vi "Process.vi"(8 "error in":errorcluster, 11 "Instrument":refnum<class "Instrument.lvclass">) -> (0 "error out":errorcluster, 3 "Instrument out":refnum<class "Instrument.lvclass">)   [LabVIEW 2016, in "Instrument.lvclass"]
doc: "---------------------------------------------------------------\nJKI State Machine Objects™\nhttp://jki.net/state-machine-objects/\nCopyright (C) 2005-2015, JKI <info@jki.net>\nALL RIGHTS RESERVED"
uses:
  Instrument.lvclass
  C:/Program Files (x86)/National Instruments/LabVIEW 2016/vi.lib/JKI/JKI SMO/SMO/SMO.lvclass
  <vilib>/JKI/JKI SMO/SMO/Typedefs/Parent Call--Enum.ctl
  RemoteControl/Typedefs/Message--Cluster.ctl
  RemoteControl/Typedefs/PrivateEvents--RemoteControl.Configure.ctl
  Logger.PGSQL/Typedefs/PrivateEvents--Logger.PGSQL.Write Variable.ctl
  <vilib>/JKI/JKI SMO/SMO/Typedefs/Public Events.ctl
  <vilib>/JKI/JKI SMO/SMO/Typedefs/SMOState --Enum.ctl
  <vilib>/JKI/JKI SMO/SMO/Typedefs/Reserve State--Enum.ctl
  RemoteControl/Typedefs/PrivateEvents--RemoteControl.SendMessageToProcess.ctl
  RemoteControl/RemoteControl.lvclass
  Logger.Error/Logger.Error.lvclass
  Logger.PGSQL/Logger.PGSQL.lvclass
  <vilib>/JKI/JKI SMO/SMO/SMO.lvclass
panel:
  out "Local Command":string
  out "Name":string
  out "Remote Command":string
  # "1. Receives & processes commands from RemoteControl process\n2. Logs instrument settings to DSC using Logger process"
  # "INSTRUMENT"
  # "For instructions on how to use the JKI State Machine Objects, examples and video tutorials, visit:\nhttp://jki.net/state-machine-objects/\n\nJKI State Machine Objects™\nhttp://jki.net/state-machine-objects/\nCopyright (C) 2005-2015, JKI <info@jki.net>\nALL RIGHTS RESERVED"
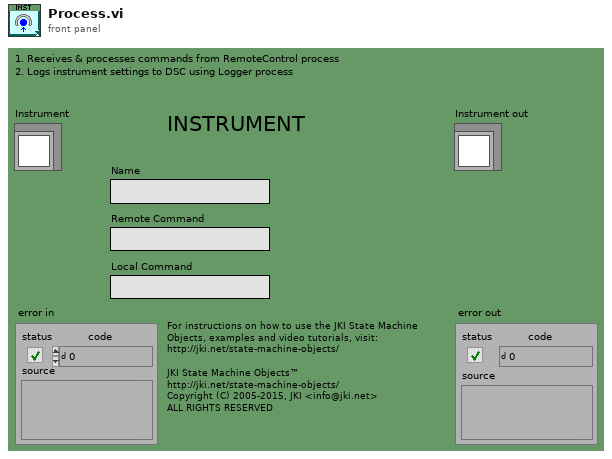
[diagram p1: front panel]
types:
  T1 = typedef "SMO.lvclass/Parent Call--Enum.ctl" = enum16{"Allows parent to run", "Does not request parent to run"}
  T2 = enum32{"invalid app kind", "Development System", "Run Time System", "Student Edition", "Embedded LabVIEW", "Evaluation", "Custom"}
  T3 = enum32{"Invalid", "Standard", "Closed", "Hidden", "Minimized", "Maximized"}
  T4 = enum32{"Bad", "Idle", "Run top level", "Running"}
  T5 = typedef "RemoteControl.lvclass/PrivateEvents--RemoteControl.SendMessageToProcess.ctl" = cluster{"Message":T6}
  T6 = typedef "RemoteControl.lvclass/Message--Cluster.ctl" = cluster{"Command":string, "Data":variant, "Message ID":i32}
  T7 = typedef "Instrument.lvclass/Dependencies--Cluster.ctl" = cluster{"RemoteControl":refnum<class "RemoteControl.lvclass">, "Logger.Error":refnum<class "Logger.Error.lvclass">, "Logger.PGSQL":refnum<class "Logger.PGSQL.lvclass">}
  T8 = typedef "RemoteControl.lvclass/PrivateEvents--RemoteControl.Configure.ctl" = cluster{"address":string, "Port":u16, "AllowedRemote":string, "Commands":string[]}
  T9 = typedef "Logger.PGSQL.lvclass/PrivateEvents--Logger.PGSQL.Write Variable.ctl" = cluster{"Address":string, "Data":variant}
  T10 = cluster{"Core":cluster{"Current VI Reference":refnum<vi>, "Close Panel on Exit?":bool, "error":errorcluster}, "Self Reference":refnum<class "Instrument.lvclass">, "Dependencies":T7, "RC Configuration":T8, "Message":T6, "getAll":variant, "Debug Mode?":bool, "PGSQL":T9}
  T11 = typedef "SMO.lvclass/SMOState --Enum.ctl" = enum16{"unknown", "Created", "Started", "Stopped"}
  T12 = cluster{"Current VI Reference":refnum<vi>, "Close Panel on Exit?":bool, "error":errorcluster}
  T13 = typedef "SMO.lvclass/Public Events.ctl" = cluster{"Error":refnum<user-event>, "State":refnum<user-event>, "Reserve State":refnum<user-event>}
  T14 = typedef "SMO.lvclass/Protected Events.ctl" = cluster{"StopProcesses":refnum<user-event>, "AbortProcesses":refnum<user-event>, "Config Changed":refnum<user-event>, "Dependency":refnum<user-event>}
  T15 = typedef "RemoteControl.lvclass/PublicEvents--Cluster.ctl" = cluster{"SendMessageFromProcess":refnum<user-event>}
  T16 = typedef "Instrument.lvclass/PrivateEvents--Cluster.ctl" = cluster{"MessageToProcess":refnum<user-event>, "Log PGSQL":refnum<user-event>}
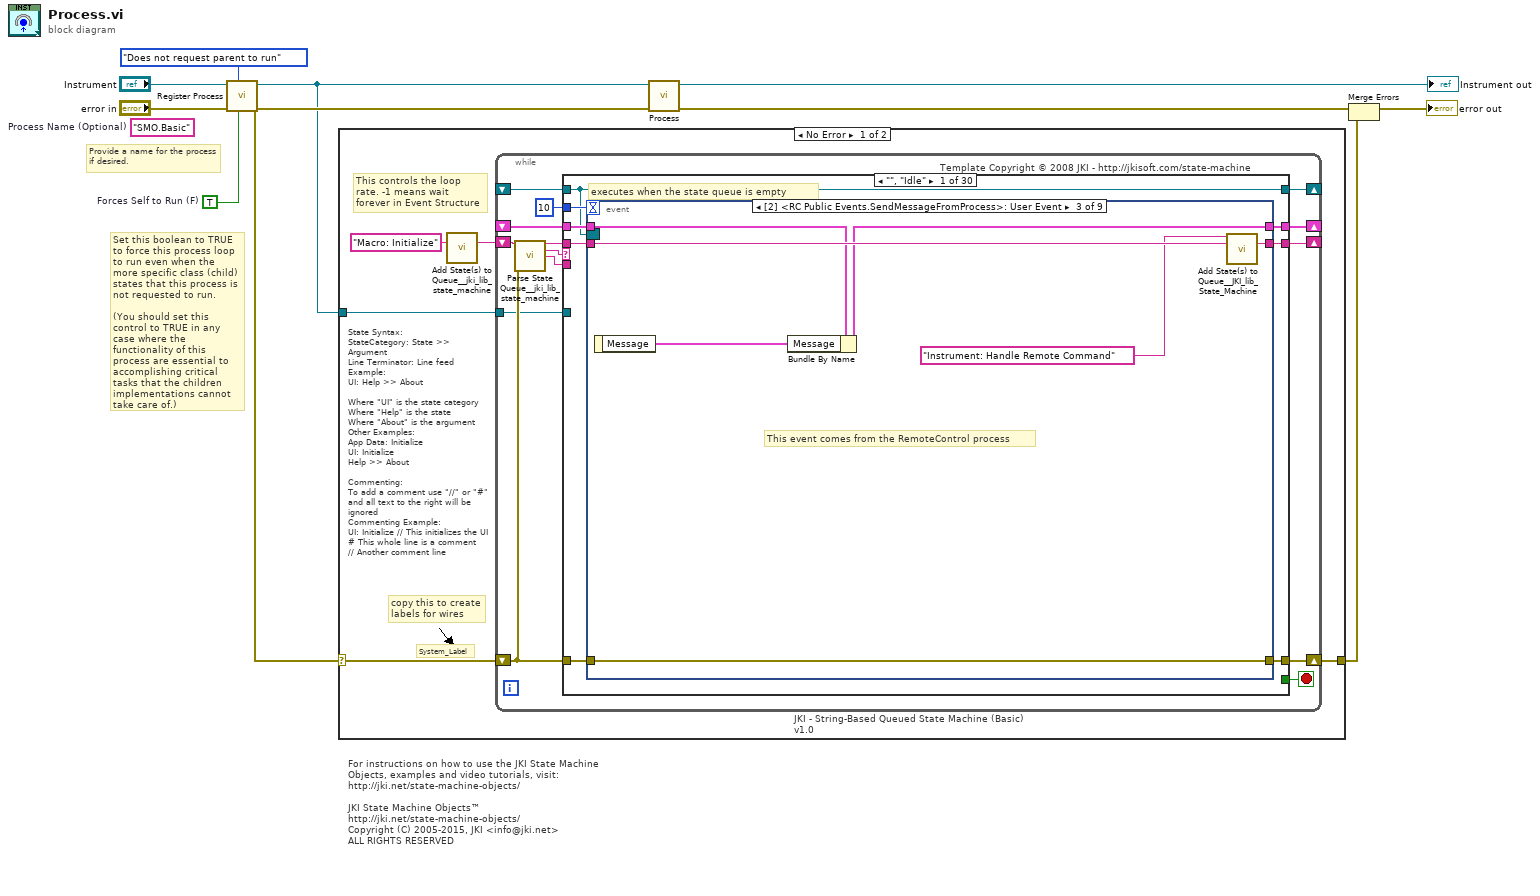
[diagram p0: block diagram]
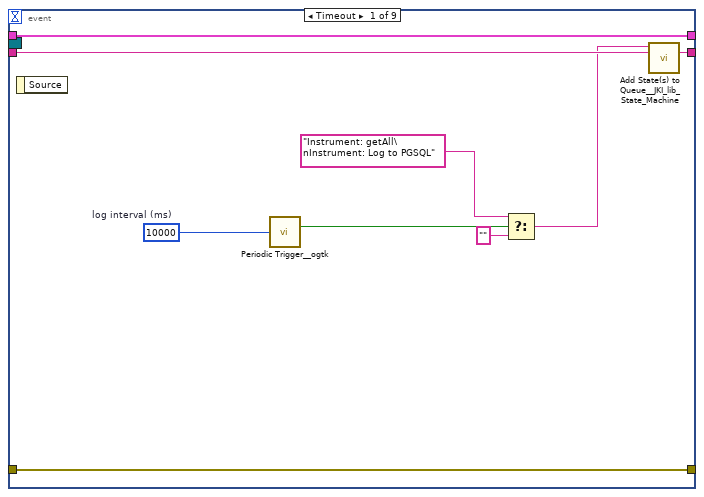
[diagram p2: hidden frame]
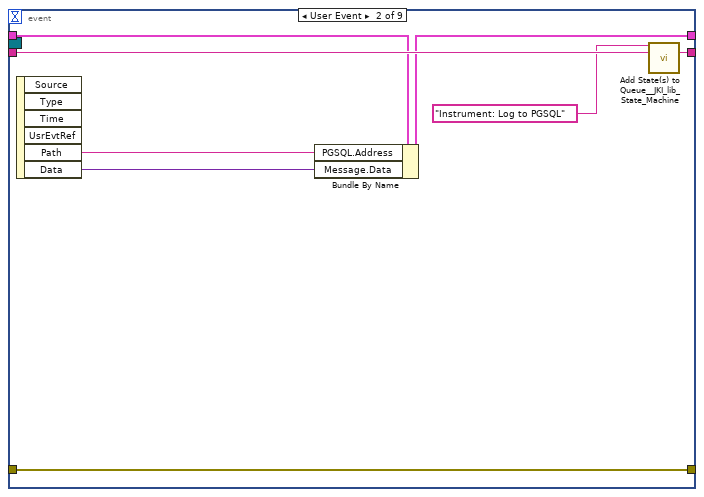
[diagram p3: hidden frame]
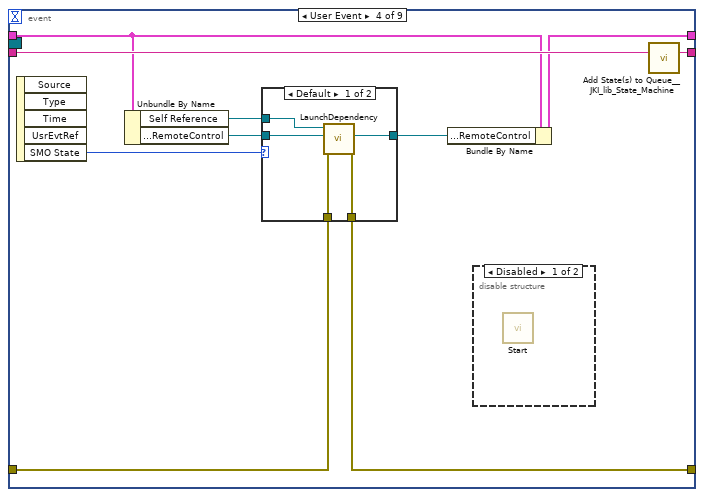
[diagram p4: hidden frame]
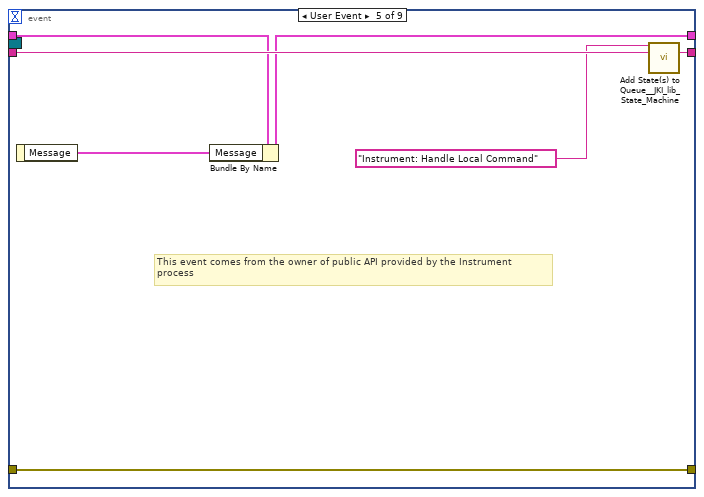
[diagram p7: hidden frame]
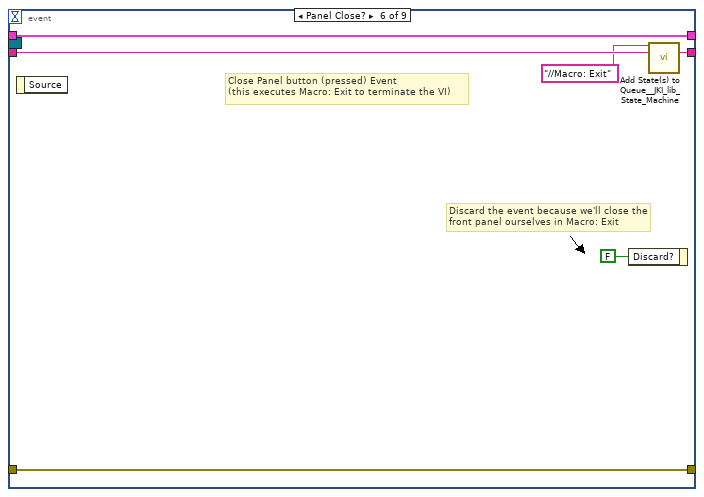
[diagram p8: hidden frame]
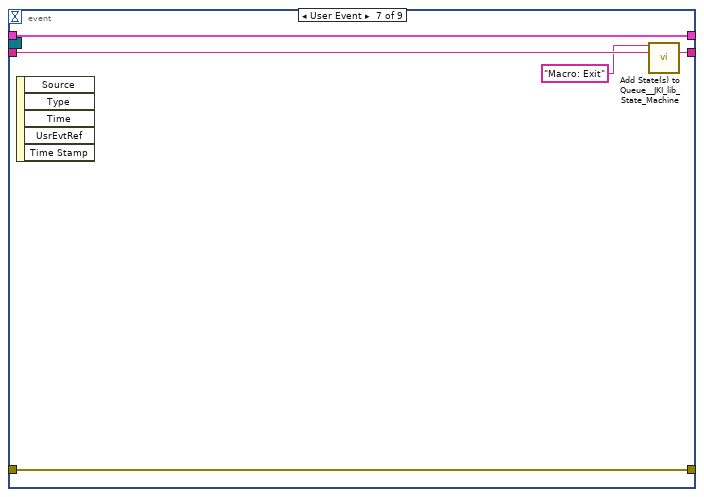
[diagram p9: hidden frame]
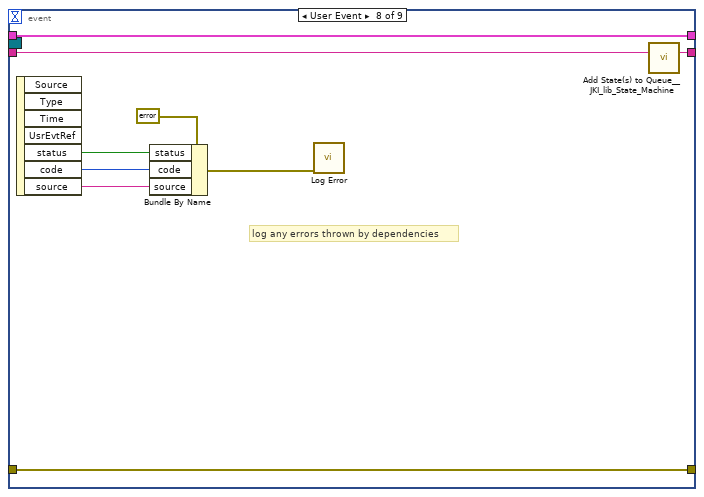
[diagram p10: hidden frame]
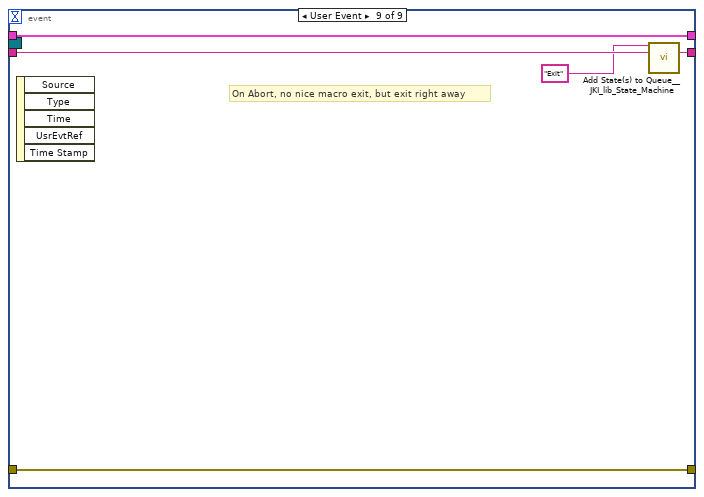
[diagram p11: hidden frame]
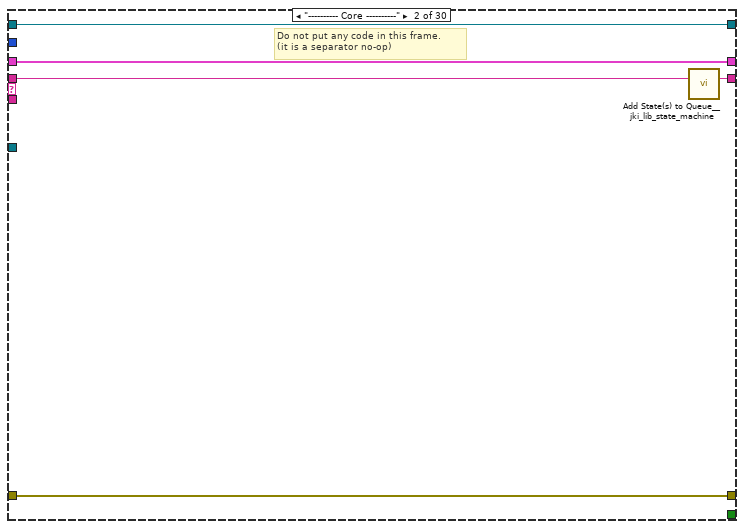
[diagram p12: hidden frame]
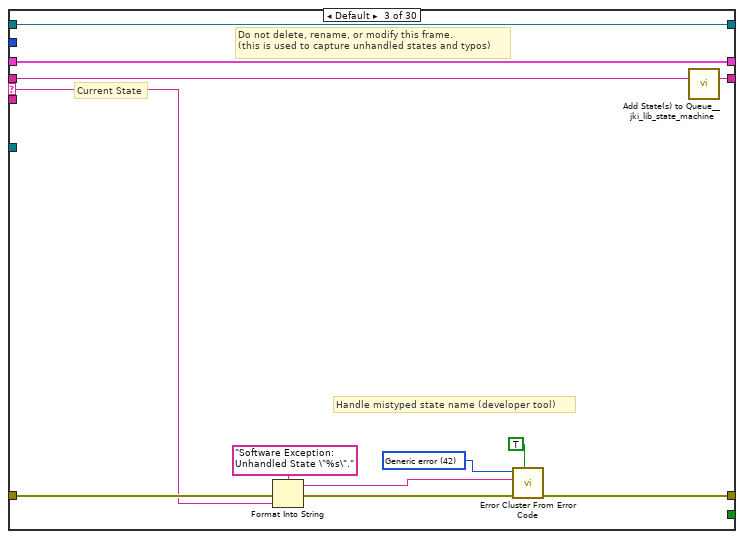
[diagram p13: hidden frame]
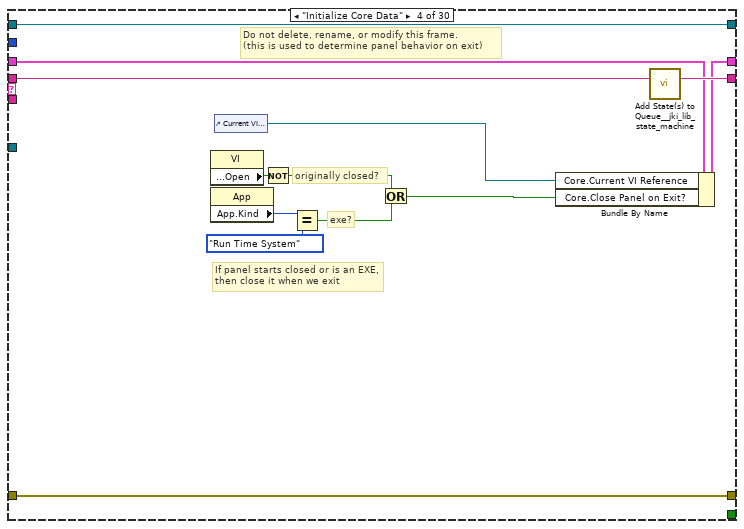
[diagram p14: hidden frame]
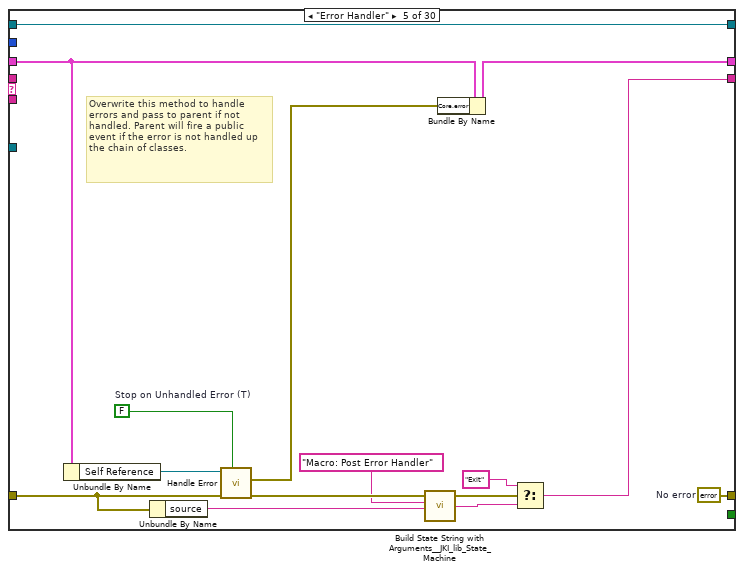
[diagram p15: hidden frame]
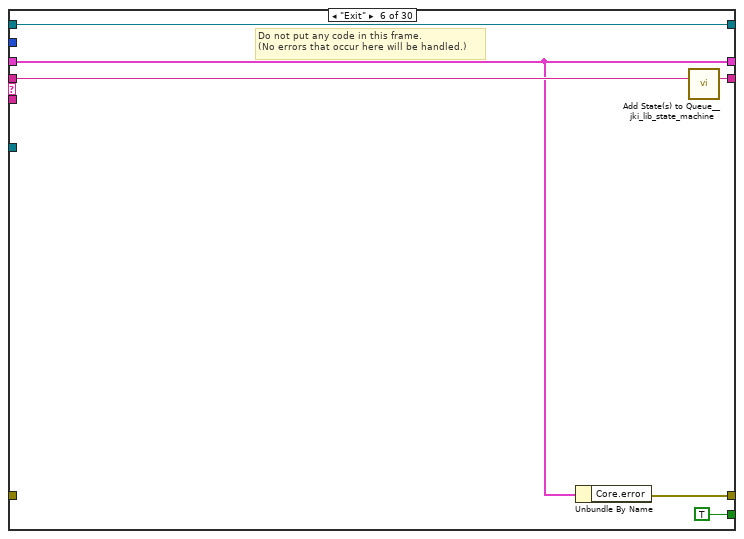
[diagram p16: hidden frame]
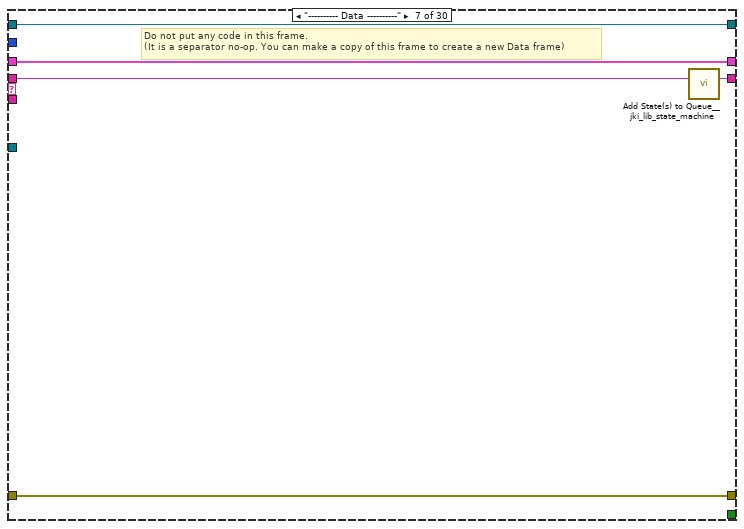
[diagram p17: hidden frame]
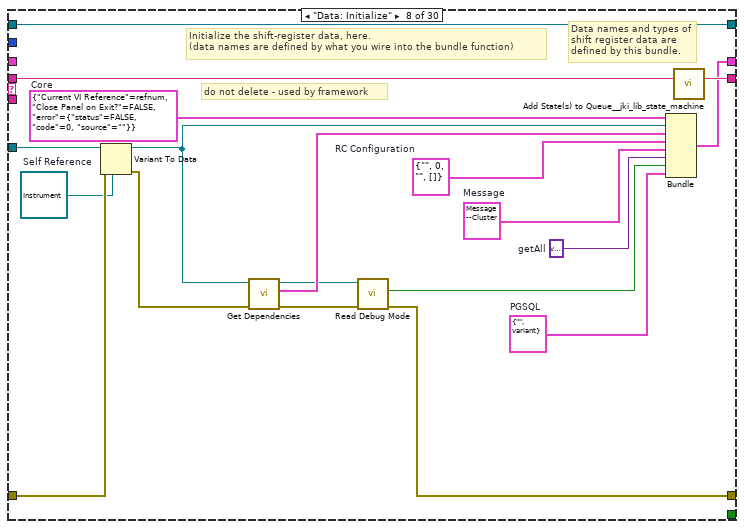
[diagram p18: hidden frame]
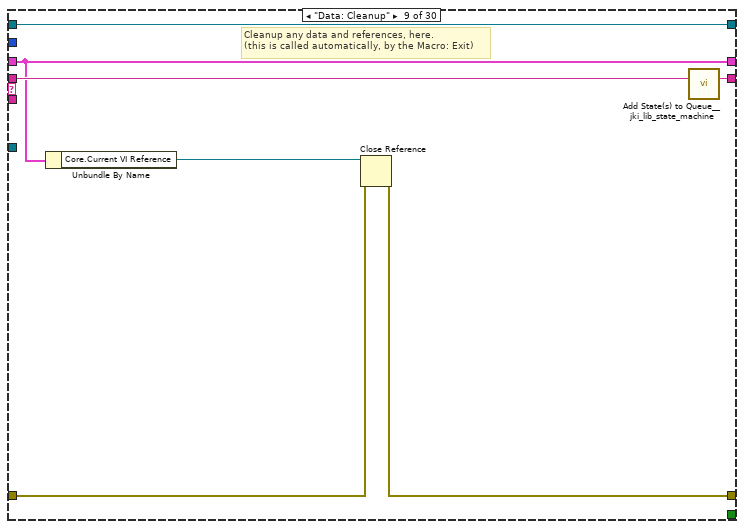
[diagram p19: hidden frame]
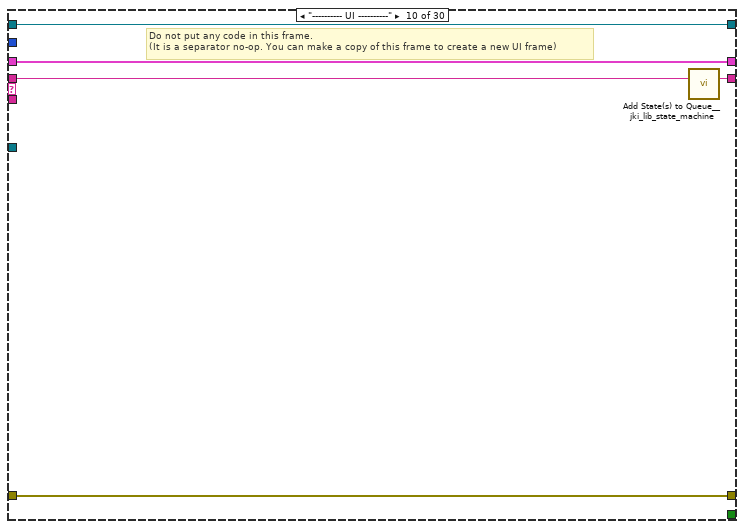
[diagram p20: hidden frame]
diagram:
  w1 = TRUE  # Forces Self to Run (F)
  (unwired) "SMO.Basic"  # Process Name (Optional)
  # "Provide a name for the process\nif desired."
  # "Set this boolean to TRUE to force this process loop to run even when the more specific class (child) states that this process is not requested to run.\n\n(You should set this control to TRUE in any case where the functionality of this process are essential to accomplishing critical tasks that the children implementations cannot take care of.)"
  # "For instructions on how to use the JKI State Machine Objects, examples and video tutorials, visit:\nhttp://jki.net/state-machine-objects/\n\nJKI State Machine Objects™\nhttp://jki.net/state-machine-objects/\nCopyright (C) 2005-2015, JKI <info@jki.net>\nALL RIGHTS RESERVED"
  n1 = call <vilib>:"Register Process.vi"("Forces Self to Run (F)"=w1, "Parent Call"=Parent_Call--Enum."Does not request parent to run", "error in (no error)"="error in", "SMO"="Instrument") -> ("error out"=w7:errorcluster, "SMO out"=w6:refnum<class "Instrument.lvclass">)  [unwired: 6 in]
  n2 = case shown="No Error" w7 {
    selector: w7 -> [w12 w487]
    tunnel: w6 -> [w13 _]
    tunnel: [w11 w487] -> w3
    frame No Error {
      # "State Syntax:\nStateCategory: State >> Argument\nLine Terminator: Line feed\nExample:\nUI: Help >> About\n\nWhere \"UI\" is the state category\nWhere \"Help\" is the state\nWhere \"About\" is the argument\nOther Examples:\nApp Data: Initialize\nUI: Initialize\nHelp >> About\n\nCommenting:\nTo add a comment use \"//\" or \"#\" and all text to the right will be ignored\nCommenting Example:\nUI: Initialize // This initializes the UI\n# This whole line is a comment\n// Another comment line"
      # "copy this to create labels for wires"
      # "This controls the loop rate. -1 means wait forever in Event Structure"
      # "System_Label"
      n3 = call <vilib>:"Add State(s) to Queue__jki_lib_state_machine.vi"("State(s) in (\"\")"="Macro: Initialize") -> ("States Out"=w15:string)  [unwired: 14 in]
      n4 = while "JKI - String-Based Queued State Machine (Basic) v1.0" {
        shift-right: [w22] -> _
        shift-left: _ -> [w21]
        shift-right: [w25] -> w11
        shift-left: w12 -> [w19]
        shift-right: [w24] -> _
        shift-left: w15 -> [w26]
        tunnel: w13 -> [w16]
        shift-right: [w18] -> _
        shift-left: _ -> [w17]
        stop <- w23 stop-if-true
        # "Template Copyright © 2008 JKI - http://jkisoft.com/state-machine"
        n5 = call <vilib>:"Parse State Queue__jki_lib_state_machine.vi"("State Queue"=w26, "Error In (no error)"=w19) -> ("Remaining States"=w28:string, "Current State"=w29:string, "Arguments"=w27:string)  [unwired: 11 in]
        n6 = case shown="\"\", \"Idle\"" w29 {
          selector: w29 -> [_ _ w117 _ _ _ _ _ _ _ _ _ _ _ _ _ _ _ _ _ _ _ _ _ _ _ _ _ _ _]
          tunnel: w28 -> [w37 w115 w121 w140 _ w160 w165 w184 w191 w196 w204 w211 w227 w264 w269 w293 w312 _ w329 w340 w345 w379 w385 w390 w404 w428 w449 w468 w477 w486]
          tunnel: w27 -> [_ _ _ _ _ _ _ _ _ _ _ w205 w221 _ _ _ _ w314 _ _ _ _ _ _ _ _ _ _ _ _]
          tunnel: w21 -> [w35 w112 w119 w131 w151 w156 w162 _ w186 w193 w201 w209 w223 w259 w266 w274 w304 w316 w326 w337 w342 w377 w383 w388 w396 w423 w439 w462 w470 w479]
          tunnel: [w34 w113 w123 w137 w152 w155 w163 w168 w187 w194 w197 w206 w224 w260 w267 w270 w310 w317 w327 w331 w343 w374 w381 w386 w394 w421 w443 w463 w472 w481] -> w25
          tunnel: w19 -> [w33 w113 w122 w137 w144 _ w163 w181 w188 w194 w198 w207 w225 w261 w267 w271 w310 w317 w327 w332 w343 w372 w381 w386 w400 w425 w446 w464 w474 w483]
          tunnel: [w36 w114 w120 w139 w147 w159 w164 w183 w190 w195 w203 w210 w226 w263 w268 w292 w311 w323 w328 w339 w344 w378 w384 w389 w403 w427 w448 w467 w476 w485] -> w24
          tunnel: [_ _ _ _ _ TRUE _ _ _ _ _ _ _ _ _ _ _ _ _ _ _ _ _ _ _ _ _ _ _ _] -> w23
          tunnel: [w32 w112 w119 w138 w150 w156 w162 w182 w186 w193 w201 w209 w223 w259 w266 w274 w304 w316 w326 w337 w342 w377 w383 w388 w396 w423 w438 w462 w469 w478] -> w22
          tunnel: 10 ("Timeout") -> [w31 _ _ _ _ _ _ _ _ _ _ _ _ _ _ _ _ _ _ _ _ _ _ _ _ _ _ _ _ _]
          tunnel: [w30 w111 w116 w128 w154 w157 w161 w179 w185 w192 w202 w208 w220 w262 w265 w291 w305 w324 w325 w338 w341 w376 w382 w387 w402 w426 w447 w466 w475 w484] -> w18
          tunnel: w17 -> [w30 w111 w116 w128 w154 w157 w161 w179 w185 w192 w202 w208 w220 w262 w265 w291 w305 w324 w325 w338 w341 _ w382 w387 w402 w426 w447 w466 w475 w484]
          tunnel: w16 -> [_ _ _ _ _ _ _ w176 _ _ _ _ _ _ _ w273 _ _ _ _ _ _ _ _ _ _ _ _ _ _]
          frame "", "Idle" {
            # "executes when the state queue is empty"
            n7 = event shown="[2] <RC Public Events.SendMessageFromProcess>: User Event" {
              selector: w30 -> [_ _ _ _ _ _ _ _ _]
              dyn-events: _ -> [_ _ _ _ _ _ _ _ _]
              timeout: w31 -> [_ _ _ _ _ _ _ _ _]
              tunnel: w37 -> [w46 w54 w61 w71 w85 w91 w96 w105 w110]
              tunnel: [w45 w53 w60 w70 w84 w90 w95 w104 w109] -> w36
              tunnel: w35 -> [w39 w49 w58 w63 w82 w88 w93 w102 w107]
              tunnel: [w44 w52 w59 w66 w83 w89 w94 w103 w108] -> w34
              tunnel: w33 -> [w44 w52 w59 w67 w83 w89 w94 w103 w108]
              tunnel: [w39 w48 w57 w62 w81 w88 w93 w102 w107] -> w32
              event Timeout {
                w40 = u32 10000  # log interval (ms)
                n8 = event-data() -> ()  [unwired: 1 in, 1 out]
                n9 = call <userlib>:"Periodic Trigger__ogtk.vi"("time (ms)"=w40) -> ("Triggered"=w42:bool)  [unwired: 12 in, 2 out]
                n10 = Select(t="Instrument: getAll\nInstrument: Log to PGSQL" ("State(s) in Front (\"\")"), s=w42, f="") -> (s? t:f=w43:string)
                n11 = call <vilib>:"Add State(s) to Queue__JKI_lib_State_Machine.vi"("State(s) in Front (\"\")"=w43, "State(s) in (\"\")"=w46) -> ("States Out"=w45:string)  [unwired: 13 in]
              }
              event User Event {
                n12 = event-data() -> ("Path"=w51:string, "Data"=w50:variant)  [unwired: 1 in, 4 out]
                n13 = Bundle By Name(cluster=w49, "PGSQL.Address"=w51, "Message.Data"=w50) -> (w48:T10)
                n14 = call <vilib>:"Add State(s) to Queue__JKI_lib_State_Machine.vi"("State(s) in Front (\"\")"="Instrument: Log to PGSQL" ("State(s) in Front (\"\")"), "State(s) in (\"\")"=w54) -> ("States Out"=w53:string)  [unwired: 13 in]
              }
              event User Event {
                # "This event comes from the RemoteControl process"
                n15 = event-data() -> ("Message"=w56:T6)  [unwired: 1 in]
                n16 = Bundle By Name(cluster=w58, "Message"=w56) -> (w57:T10)
                n17 = call <vilib>:"Add State(s) to Queue__JKI_lib_State_Machine.vi"("State(s) in Front (\"\")"="Instrument: Handle Remote Command" ("State(s) in Front (\"\")"), "State(s) in (\"\")"=w61) -> ("States Out"=w60:string)  [unwired: 13 in]
              }
              event User Event {
                n18 = event-data() -> ("SMO State"=w69:T11)  [unwired: 1 in, 4 out]
                n19 = Unbundle By Name(w63) -> ("Self Reference"=w65:refnum<class "Instrument.lvclass">, "Dependencies.RemoteControl"=w68:refnum<class "RemoteControl.lvclass">)
                n20 = case shown="Default" w69 {
                  tunnel: w68 -> [w73 w77]
                  tunnel: w67 -> [w76 w78]
                  tunnel: [w75 w78] -> w66
                  tunnel: w65 -> [w74 _]
                  tunnel: [w72 w77] -> w64
                  frame Default {
                    n21 = call <vilib>:"LaunchDependency.vi"("error in (no error)"=w76, "Dependency Type"=w73, "SMO in"=w74) -> ("error out"=w75:errorcluster, "Dependency Reference"=w72:refnum<class "RemoteControl.lvclass">)  [unwired: 5 in, 2 out]
                  }
                  frame "Started" {
                  }
                }
                n22 = Bundle By Name(cluster=w63, "Dependencies.RemoteControl"=w64) -> (w62:T10)
                n23 = disable-structure shown="Disabled" {
                  frame Disabled {
                    n24 = call <vilib>:"Start.vi"() -> ()  [unwired: 10 in, 2 out]
                  }
                  frame Enabled {
                  }
                }
                n25 = call <vilib>:"Add State(s) to Queue__JKI_lib_State_Machine.vi"("State(s) in (\"\")"=w71) -> ("States Out"=w70:string)  [unwired: 14 in]
              }
              event User Event {
                # "This event comes from the owner of public API provided by the Instrument\nprocess"
                n26 = event-data() -> ("Message"=w80:T6)  [unwired: 1 in]
                n27 = Bundle By Name(cluster=w82, "Message"=w80) -> (w81:T10)
                n28 = call <vilib>:"Add State(s) to Queue__JKI_lib_State_Machine.vi"("State(s) in Front (\"\")"="Instrument: Handle Local Command" ("State(s) in Front (\"\")"), "State(s) in (\"\")"=w85) -> ("States Out"=w84:string)  [unwired: 13 in]
              }
              event Panel Close? {
                # "Discard the event because we'll close the front panel ourselves in Macro: Exit"
                # "Close Panel button (pressed) Event\n(this executes Macro: Exit to terminate the VI)"
                n29 = event-data() -> ()  [unwired: 1 in, 1 out]
                n30 = event-data("Discard?"=FALSE) -> ()  [unwired: 1 in, 1 out]
                n31 = call <vilib>:"Add State(s) to Queue__JKI_lib_State_Machine.vi"("State(s) in Front (\"\")"="//Macro: Exit", "State(s) in (\"\")"=w91) -> ("States Out"=w90:string)  [unwired: 13 in]
              }
              event User Event {
                n32 = event-data() -> ()  [unwired: 1 in, 5 out]
                n33 = call <vilib>:"Add State(s) to Queue__JKI_lib_State_Machine.vi"("State(s) in Front (\"\")"="Macro: Exit", "State(s) in (\"\")"=w96) -> ("States Out"=w95:string)  [unwired: 13 in]
              }
              event User Event {
                # "log any errors thrown by dependencies"
                n34 = event-data() -> ("status"=w100:bool, "code"=w101:i32, "source"=w99:string)  [unwired: 1 in, 4 out]
                n35 = Bundle By Name(cluster=errorcluster {"status"=FALSE, "code"=0, "source"=""} ("error in"), "status"=w100, "code"=w101, "source"=w99) -> (w97:errorcluster)
                n36 = call "Log Error.vi"("error in (no error)"=w97) -> ()  [unwired: 9 in, 2 out]
                n37 = call <vilib>:"Add State(s) to Queue__JKI_lib_State_Machine.vi"("State(s) in (\"\")"=w105) -> ("States Out"=w104:string)  [unwired: 14 in]
              }
              event User Event {
                # "On Abort, no nice macro exit, but exit right away"
                n38 = event-data() -> ()  [unwired: 1 in, 5 out]
                n39 = call <vilib>:"Add State(s) to Queue__JKI_lib_State_Machine.vi"("State(s) in Front (\"\")"="Exit", "State(s) in (\"\")"=w110) -> ("States Out"=w109:string)  [unwired: 13 in]
              }
            }
          }
          frame "---------- Core ----------" {
            # "Do not put any code in this frame.\n(it is a separator no-op)"
            n40 = call <vilib>:"Add State(s) to Queue__jki_lib_state_machine.vi"("State(s) in (\"\")"=w115) -> ("States Out"=w114:string)  [unwired: 14 in]
          }
          frame Default {
            w126 = 42 items=["No error", "Argument error", "Memory is full", "Out of zone", "End of file", "File already open", "Generic file I/O error", "File not found", "File permission error", "Disk is full", "Duplicate path", "Too many files open", "System feature not enabled", "Resource file not found", "Cannot add resource", "Resource not found", "Image not found", "Image memory error", "Pen does not exist", "Config type invalid", "Config token not found", "Config parse error", "Config memory error", "Bad external code format", "Bad external code offset", "External code not present", "Null window", "Destroy window error", "Null menu", "Print aborted", "Bad print record", "Print driver error", "Windows error during printing", "Memory error during printing", "Print dialog error", "Generic print error", "Invalid device refnum", "Device not found", "Device parameter error", "Device unit error", "Cannot open device", "Device call aborted", "Generic error", "Cancelled by user", "Object ID too low", "Object ID too high", "Object not in heap", "Unknown heap", "Unknown object (invalid DefProc)", "Unknown object (DefProc not in table)", "Message out of range", "Invalid (null) method", "Unknown message", "Manager call not supported", "Bad address", "Network operation in progress", "Network operation timed out", "Connection is busy", "Network attribute not supported", "Network error", "Address in use", "System out of memory", "Connection aborted", "Connection refused", "Not connected", "Already connected", "Connection closed", "Initialization error (interapplication manager)", "Bad occurrence", "Wait on unbound occurrence handler", "Occurrence queue overflow", "Datalog type conflict", "Unused", "Unrecognized type (interapplication manager)", "Memory corrupt", "Failed to make temporary DLL", "Old CIN version", "Drag socket not found", "Failed to load drop-object", "Failed to register OLE object", "Failed to release OLE object", "Format specifier type mismatch", "Unknown format specifier", "Too few format specifiers", "Too many format specifiers", "Scan failed", "Newer CIN version", "Error converting to variant", "Runtime menu error", "Password tampered", "Variant attribute not found", "Incompatible variant data type", "Event data is not available", "Event Store is not present", "Occurrence is not found", "Event Queue is not created", "Event info is not available", "Refnum passed is NULL", "Error retrieving Class GUID", "Error retrieving CoClass GUID", "Error retrieving TypeLib GUID.", "Bad built application magic bytes.", "Specific driver is different from the specific driver associated with the Logical Name.", "There is no session opened to the class driver.", "Max Error", "MAX - Error with config objects", "MAX - Error loading configuration", "MAX - Group not supported"]
            # "Current State"
            # "Do not delete, rename, or modify this frame.\n(this is used to capture unhandled states and typos)"
            # "Handle mistyped state name (developer tool)"
            n41 = Format Into String(format string="Software Exception: Unhandled State \"%s\"." ("message"), error in=w122, w117) -> (resulting string=w125:string, error out=w124:errorcluster)  [unwired: 1 in]
            n42 = call <vilib>:"Error Cluster From Error Code.vi"("show call chain? (False)"=TRUE, "error in (no error)"=w124, "error message (\"\")"=w125, "error code (0)"=w126) -> ("error out"=w123:errorcluster)  [unwired: 5 in]
            n43 = call <vilib>:"Add State(s) to Queue__jki_lib_state_machine.vi"("State(s) in (\"\")"=w121) -> ("States Out"=w120:string)  [unwired: 14 in]
          }
          frame "Initialize Core Data" {
            # "Do not delete, rename, or modify this frame.\n(this is used to determine panel behavior on exit)"
            # "originally closed?"
            # "exe?"
            # "If panel starts closed or is an EXE, then close it when we exit"
            n44 = property class="VI"() -> ("Front Panel.Open"=w136:bool)  [unwired: 2 in, 2 out]
            n45 = property class="App"() -> ("App.Kind"=w135:T2)  [unwired: 2 in, 2 out]
            n46 = control-ref of="Current VI Reference"() -> (w129:refnum<vi>)
            n47 = Not(x=w136) -> (.not. x?=w133:bool)
            n48 = Equal?(x=w135, y=T2."Run Time System" ("Application:Kind")) -> (x = y?=w132:bool)
            n49 = Or(x=w133, y=w132) -> (x .or. y?=w130:bool)
            n50 = Bundle By Name(cluster=w131, "Core.Current VI Reference"=w129, "Core.Close Panel on Exit?"=w130) -> (w138:T10)
            n51 = call <vilib>:"Add State(s) to Queue__jki_lib_state_machine.vi"("State(s) in (\"\")"=w140) -> ("States Out"=w139:string)  [unwired: 14 in]
          }
          frame "Error Handler" {
            w148 = FALSE  # Stop on Unhandled Error (T)
            w152 = errorcluster {"status"=FALSE, "code"=0, "source"=""}  # No error
            # "Overwrite this method to handle errors and pass to parent if not handled. Parent will fire a public event if the error is not handled up the chain of classes."
            n52 = Unbundle By Name(w151) -> ("Self Reference"=w153:refnum<class "Instrument.lvclass">)
            n53 = Unbundle By Name(w144) -> ("source"=w143:string)
            n54 = call-dynamic "Handle Error.vi"("Stop on Unhandled Error (T)"=w148, "error in"=w144, "Instrument"=w153) -> ("handling error"=w145:errorcluster, "Unhandled error"=w146:errorcluster)  [unwired: 6 in, 1 out]
            n55 = call <vilib>:"Build State String with Arguments__JKI_lib_State_Machine.vi"("Arguments (\"\")"=w143, "State"="Macro: Post Error Handler") -> ("State with Arguments"=w142:string)  [unwired: 4 in]
            n56 = Bundle By Name(cluster=w151, "Core.error"=w146) -> (w150:T10)
            n57 = Select(t="Exit", s=w145, f=w142) -> (s? t:f=w147:string)
          }
          frame "Exit" {
            # "Do not put any code in this frame.\n(No errors that occur here will be handled.)"
            n58 = Unbundle By Name(w156) -> ("Core.error"=w155:errorcluster)
            n59 = call <vilib>:"Add State(s) to Queue__jki_lib_state_machine.vi"("State(s) in (\"\")"=w160) -> ("States Out"=w159:string)  [unwired: 14 in]
          }
          frame "---------- Data ----------" {
            # "Do not put any code in this frame.\n(It is a separator no-op. You can make a copy of this frame to create a new Data frame)"
            n60 = call <vilib>:"Add State(s) to Queue__jki_lib_state_machine.vi"("State(s) in (\"\")"=w165) -> ("States Out"=w164:string)  [unwired: 14 in]
          }
          frame "Data: Initialize" {
            w166 = T9 {"Address"="", "Data"=variant}  # PGSQL
            w173 = variant  # getAll
            w174 = T8 {"address"="", "Port"=0, "AllowedRemote"="", "Commands"=[]}  # RC Configuration
            w175 = T6 {"Command"="", "Data"=variant, "Message ID"=0}  # Message
            w178 = T12 {"Current VI Reference"=refnum, "Close Panel on Exit?"=FALSE, "error"={"status"=FALSE, "code"=0, "source"=""}}  # Core
            w180 = refnum<class "Instrument.lvclass"> refnum  # Self Reference
            # "do not delete - used by framework"
            # "Data names and types of shift register data are defined by this bundle."
            # "Initialize the shift-register data, here.\n(data names are defined by what you wire into the bundle function)"
            n61 = Variant To Data(error in=w181, type=w180, Variant=w176) -> (data=w171:refnum<class "Instrument.lvclass">, error out=w177:errorcluster)
            n62 = call "Get Dependencies.vi"("error in (no error)"=w177, "Instrument in"=w171) -> ("error out"=w169:errorcluster, "Dependencies"=w172:T7, "SMO out"=w170:refnum<class "Instrument.lvclass">)  [unwired: 7 in]
            n63 = call-dynamic "Read Debug Mode.vi"("error in (no error)"=w169, "Instrument in"=w170) -> ("error out"=w168:errorcluster, "Debug Mode?"=w167:bool)  [unwired: 7 in, 1 out]
            n64 = Bundle("Core"=w178, "Self Reference"=w171, "Dependencies"=w172, "RC Configuration"=w174, "Message"=w175, "getAll"=w173, "Debug Mode?"=w167, "PGSQL"=w166) -> (w182:T10)  [unwired: 1 in]
            n65 = call <vilib>:"Add State(s) to Queue__jki_lib_state_machine.vi"("State(s) in (\"\")"=w184) -> ("States Out"=w183:string)  [unwired: 14 in]
          }
          frame "Data: Cleanup" {
            # "Cleanup any data and references, here.\n(this is called automatically, by the Macro: Exit)"
            n66 = Unbundle By Name(w186) -> ("Core.Current VI Reference"=w189:refnum<vi>)
            n67 = Close Reference(reference=w189, error in (no error)=w188) -> (error out=w187:errorcluster)
            n68 = call <vilib>:"Add State(s) to Queue__jki_lib_state_machine.vi"("State(s) in (\"\")"=w191) -> ("States Out"=w190:string)  [unwired: 14 in]
          }
          frame "---------- UI ----------" {
            # "Do not put any code in this frame.\n(It is a separator no-op. You can make a copy of this frame to create a new UI frame)"
            n69 = call <vilib>:"Add State(s) to Queue__jki_lib_state_machine.vi"("State(s) in (\"\")"=w196) -> ("States Out"=w195:string)  [unwired: 14 in]
          }
          frame "UI: Initialize" {
            # "Initialize the User Interface, here.\n(this is called automatically, by the Macro: Init)"
            n70 = Unbundle By Name(w201) -> ("Self Reference"=w200:refnum<class "Instrument.lvclass">)
            n71 = call <vilib>:"GetName.vi"("error in (no error)"=w198, "SMO"=w200) -> ("error out"=w197:errorcluster, "Name"=→"Name":string)  [unwired: 7 in, 1 out]
            n72 = call <vilib>:"Add State(s) to Queue__jki_lib_state_machine.vi"("State(s) in (\"\")"=w204) -> ("States Out"=w203:string)  [unwired: 14 in]
          }
          frame "UI: Cursor Set" {
            # "Argument"
            # "Initialize the User Interface, here.\n(this is called automatically, by the Macro: Init)"
            n73 = disable-structure shown="Default" {
              disable-tunnel: w207 -> [w212 w215]
              disable-tunnel: [w212 w214] -> w206
              disable-tunnel: w205 -> [_ w213]
              frame condition #0 {
              }
              frame condition #1 (active) {
                n74 = case shown="\"Busy\"" w213 {
                  tunnel: w215 -> [w217 w219]
                  tunnel: [w216 w218] -> w214
                  frame "Idle", Default {
                    n75 = call <vilib>:"Unset Busy.vi"("error in (no error)"=w217) -> ("error out"=w216:errorcluster)  [unwired: 10 in]
                  }
                  frame "Busy" {
                    n76 = call <vilib>:"Set Busy.vi"("error in (no error)"=w219) -> ("error out"=w218:errorcluster)  [unwired: 9 in, 1 out]
                  }
                }
              }
            }
            n77 = call <vilib>:"Add State(s) to Queue__jki_lib_state_machine.vi"("State(s) in (\"\")"=w211) -> ("States Out"=w210:string)  [unwired: 14 in]
          }
          frame "UI: Front Panel State" {
            # "Argument"
            # "Set Front Panel Open or Closed\n(Usage: \"UI: Front Panel State >> Open|Close\")"
            n78 = Unbundle By Name(w223) -> ("Core.Current VI Reference"=w222:refnum<vi>)
            n79 = disable-structure shown="Default" {
              disable-tunnel: w225 -> [w231 w254]
              disable-tunnel: [w230 w254] -> w224
              disable-tunnel: w222 -> [w229 _]
              disable-tunnel: w221 -> [w228 _]
              frame condition #0 (active) {
                n80 = case shown="\"Close\"" w228 {
                  tunnel: w231 -> [w235 w248]
                  tunnel: [w237 w249] -> w230
                  tunnel: w229 -> [w236 w246]
                  frame "Open", Default {
                    n81 = property class="VI"(reference=w236, error in=w235) -> (reference out=w233:refnum<vi>, error out=w234:errorcluster, "FP.State"=w232:T3)
                    n82 = case shown="Default" w232 {
                      tunnel: [w240 w243] -> w237
                      tunnel: w234 -> [w239 w243]
                      tunnel: w233 -> [w238 _]
                      frame "Closed" {
                        n83 = invoke class="VI" method="FP.Open"(reference=w238, error in=w239, "Activate"=TRUE, "State"=T3."Standard") -> (error out=w240:errorcluster)  [unwired: 1 in, 4 out]
                      }
                      frame Default {
                      }
                    }
                  }
                  frame "Close" {
                    n84 = property class="VI"(reference=w246, error in=w248) -> (reference out=w245:refnum<vi>, error out=w247:errorcluster, "FP.State"=w244:T3)
                    n85 = case shown="Default" w244 {
                      tunnel: [w250 w253] -> w249
                      tunnel: w247 -> [w250 w252]
                      tunnel: w245 -> [_ w251]
                      frame "Invalid", "Closed" {
                      }
                      frame Default {
                        n86 = invoke class="VI" method="FP.Close"(reference=w251, error in=w252) -> (error out=w253:errorcluster)  [unwired: 1 in, 2 out]
                      }
                    }
                  }
                }
              }
              frame condition #1 {
              }
            }
            n87 = call <vilib>:"Add State(s) to Queue__jki_lib_state_machine.vi"("State(s) in (\"\")"=w227) -> ("States Out"=w226:string)  [unwired: 14 in]
          }
          frame "UI: Wait" {
            n88 = Unbundle By Name(w259) -> ("Debug Mode?"=w256:bool)
            n89 = Select(t=u32 5000 ("milliseconds to wait"), s=w256, f=u32 0 ("milliseconds to wait")) -> (s? t:f=w255:u32)
            n90 = call <userlib>:"Wait (ms)__ogtk.vi"("error in (no error)"=w261, "milliseconds to wait"=w255) -> ("error out"=w260:errorcluster)  [unwired: 8 in, 1 out]
            n91 = call <vilib>:"Add State(s) to Queue__jki_lib_state_machine.vi"("State(s) in (\"\")"=w264) -> ("States Out"=w263:string)  [unwired: 14 in]
          }
          frame "---------- Macro ----------" {
            # "Do not put any code in this frame.\n(It is a separator no-op. You can make a copy of this frame to create a new Macro frame)"
            n92 = call <vilib>:"Add State(s) to Queue__jki_lib_state_machine.vi"("State(s) in (\"\")"=w269) -> ("States Out"=w268:string)  [unwired: 14 in]
          }
          frame "Macro: Initialize" {
            w283 = "Process: Sync"
            # "This needs to be called here before Data: Initialize\nto ensure that the correct argument"
            # "Initialization Macro\n(This is called once, when the VI starts)"
            n93 = control-ref of="This VI"() -> (w285:refnum<vi>)
            n94 = property class="VI"(reference=w285) -> ("Exec.State"=w284:T4)  [unwired: 1 in, 2 out]
            n95 = Equal?(x=w284, y=T4."Run top level") -> (x = y?=w289:bool)
            n96 = call-dynamic "Read Debug Mode.vi"("error in (no error)"=w271, "Instrument in"=w273) -> ("error out"=w270:errorcluster, "Debug Mode?"=w272:bool)  [unwired: 7 in, 1 out]
            n97 = Select(t="Open", s=w272, f="Close") -> (s? t:f=w276:string)
            n98 = Select(t=w283, s=w289, f="") -> ()  [unwired: 1 out]
            n99 = call <vilib>:"Build State String with Arguments__JKI_lib_State_Machine.vi"("Arguments (\"\")"=w276, "State"="UI: Front Panel State") -> ("State with Arguments"=w279:string)  [unwired: 4 in]
            n100 = call <vilib>:"Add State(s) to Queue__jki_lib_state_machine.vi"("State(s) in Front (\"\")"="UI: Initialize", "State(s) in (\"\")"=w279, "State(s) at Back (\"\")"="UI: Wait\nInstrument: Open") -> ("States Out"=w277:string)  [unwired: 12 in]
            n101 = call <vilib>:"Add State(s) to Queue__jki_lib_state_machine.vi"("State(s) in Front (\"\")"="Data: Initialize\nInitialize Core Data\nEvents: Register", "State(s) in (\"\")"=w283, "State(s) at Back (\"\")"=w277) -> ("States Out"=w286:string)  [unwired: 12 in]
            n102 = call <vilib>:"Add State(s) to Queue__jki_lib_state_machine.vi"("State(s) in Front (\"\")"=w286, "State(s) in (\"\")"=w293) -> ("States Out"=w292:string)  [unwired: 13 in]
          }
          frame "Macro: Exit" {
            w302 = "Instrument: Close\nData: Cleanup\nEvents: Unregister"  # Instrument: Close Data: Cleanup Events: Unregister
            # "Exit Macro\n(This is called once, when the VI exits)"
            n103 = Unbundle By Name(w304) -> ("Debug Mode?"=w298:bool, "Core.Close Panel on Exit?"=w309:bool)
            n104 = Select(t="Open", s=w298, f="Close") -> (s? t:f=w295:string)
            n105 = call <vilib>:"Build State String with Arguments__JKI_lib_State_Machine.vi"("Arguments (\"\")"=w295, "State"="UI: Front Panel State") -> ("State with Arguments"=w299:string)  [unwired: 4 in]
            n106 = Select(t=w299, s=w309, f="") -> (s? t:f=w307:string)
            n107 = call <vilib>:"Add State(s) to Queue__jki_lib_state_machine.vi"("State(s) in Front (\"\")"=w302, "State(s) in (\"\")"="Process: Sync", "State(s) at Back (\"\")"="Exit") -> ("States Out"=w301:string)  [unwired: 12 in]
            n108 = call <vilib>:"Add State(s) to Queue__jki_lib_state_machine.vi"("State(s) in (\"\")"=w307, "State(s) at Back (\"\")"=w301) -> ("States Out"=w306:string)  [unwired: 13 in]
            n109 = call <vilib>:"Add State(s) to Queue__jki_lib_state_machine.vi"("State(s) in Front (\"\")"=w306, "State(s) in (\"\")"=w312) -> ("States Out"=w311:string)  [unwired: 13 in]
          }
          frame "Macro: Post Error Handler" {
            n110 = Concatenate Strings(w314, "\nTry to reconnect?" ("message")) -> (w313:string)
            n111 = Two Button Dialog(message=w313, 1:"Shutdown" ("F button name (\"Cancel\")"), 2:"Reconnect" ("T button name (\"OK\")")) -> (T button?=w319:bool)
            n112 = Select(t="Instrument: Close\nInstrument: Open" ("States to Execute"), s=w319, f="Macro: Exit" ("States to Execute")) -> (s? t:f=w323:string)
          }
          frame "---------- Process ----------" {
            # "Template Separator\n(You can make a copy of, or modify, this frame)"
            n113 = call <vilib>:"Add State(s) to Queue__jki_lib_state_machine.vi"("State(s) in (\"\")"=w329) -> ("States Out"=w328:string)  [unwired: 14 in]
          }
          frame "Process: Sync" {
            n114 = Unbundle By Name(w337) -> ("Self Reference"=w333:refnum<class "Instrument.lvclass">)
            n115 = call <vilib>:"WaitOnProcessSync.vi"("error in (no error)"=w332, "SMO"=w333) -> ("error out"=w331:errorcluster, "Don't run?"=w336:bool)  [unwired: 7 in, 1 out]
            n116 = Select(t="Data: Cleanup\nEvents: Unregister\nExit", s=w336, f="") -> (s? t:f=w330:string)
            n117 = call <vilib>:"Add State(s) to Queue__jki_lib_state_machine.vi"("State(s) in Front (\"\")"=w330, "State(s) in (\"\")"=w340) -> ("States Out"=w339:string)  [unwired: 13 in]
          }
          frame "---------- Events ----------" {
            # "Template Separator\n(You can make a copy of, or modify, this frame)"
            n118 = call <vilib>:"Add State(s) to Queue__jki_lib_state_machine.vi"("State(s) in (\"\")"=w345) -> ("States Out"=w344:string)  [unwired: 14 in]
          }
          frame "Events: Register" {
            w359 = T13 {"Error"=refnum, "State"=refnum, "Reserve State"=refnum}  # RemoteControl.Public Events
            w358 = T13 {"Error"=refnum, "State"=refnum, "Reserve State"=refnum}  # Logger.PGSQL.Public Events
            w357 = T13 {"Error"=refnum, "State"=refnum, "Reserve State"=refnum}  # Logger.Error.Public Events
            n119 = Unbundle By Name(w377) -> ("Self Reference"=w367:refnum<class "Instrument.lvclass">, "Dependencies.RemoteControl"=w366:refnum<class "RemoteControl.lvclass">, "Dependencies.Logger.PGSQL"=w355:refnum<class "Logger.PGSQL.lvclass">, "Dependencies.Logger.Error"=w356:refnum<class "Logger.Error.lvclass">)
            n120 = call <vilib>:"GetProtectedEvents.vi"("SMO"=w367) -> ("error out"=w373:errorcluster, "SMO Protected Events"=w375:T14, "SMO out"=w354:refnum<class "Instrument.lvclass">)  [unwired: 8 in]
            n121 = call "RemoteControl.GetPublicEvents.vi"("RemoteControl"=w366) -> ("error out"=w370:errorcluster, "RC Public Events"=w369:T15, "RemoteControl out"=w353:refnum<class "RemoteControl.lvclass">)  [unwired: 8 in]
            n122 = call "Instrument.GetPrivateEvents.vi"("Instrument"=w354) -> ("error out"=w368:errorcluster, "Instrument Private Events"=w349:T16)  [unwired: 8 in, 1 out]
            n123 = call <vilib>:"GetPublicEvents.vi"("SMO"=w353) -> ("error out"=w365:errorcluster, "Public Events"=w350:T13)  [unwired: 8 in, 1 out]
            n124 = call <vilib>:"GetPublicEvents.vi"("SMO"=w355) -> ("error out"=w364:errorcluster, "Public Events"=w351:T13)  [unwired: 8 in, 1 out]
            n125 = Variant To Data(error in=w365, type=w359, Variant=w350) -> (data=w347:T13, error out=w360:errorcluster)
            n126 = Variant To Data(error in=w364, type=w358, Variant=w351) -> (data=w348:T13, error out=w361:errorcluster)
            n127 = call <vilib>:"GetPublicEvents.vi"("SMO"=w356) -> ("error out"=w363:errorcluster, "Public Events"=w352:T13)  [unwired: 8 in, 1 out]
            n128 = Variant To Data(error in=w363, type=w357, Variant=w352) -> (data=w346:T13, error out=w362:errorcluster)
            n129 = register-events(w375, w369, w349, w347, w348, w346) -> (reference out=w376:refnum<event-registration>, error out=w371:errorcluster)  [unwired: 2 in]
            n130 = Merge Errors(w360, w361, w362, w368, w371, w370, w373, w372) -> (w374:errorcluster)
            n131 = call <vilib>:"Add State(s) to Queue__jki_lib_state_machine.vi"("State(s) in (\"\")"=w379) -> ("States Out"=w378:string)  [unwired: 14 in]
          }
          frame "Events: Unregister" {
            n132 = Unregister For Events(event registration refnum=w382, error in=w381) -> (error out=w380:errorcluster)
            n133 = call <vilib>:"Clear Errors.vi"("error in (no error)"=w380) -> ()  [unwired: 5 in, 2 out]
            n134 = call <vilib>:"Add State(s) to Queue__jki_lib_state_machine.vi"("State(s) in (\"\")"=w385) -> ("States Out"=w384:string)  [unwired: 14 in]
          }
          frame "---------- Instrument ----------" {
            n135 = call <vilib>:"Add State(s) to Queue__jki_lib_state_machine.vi"("State(s) in (\"\")"=w390) -> ("States Out"=w389:string)  [unwired: 14 in]
          }
          frame "Instrument: Handle Remote Command" {
            # "#todo\nput driver stuff inside this one"
            # "do stuff in reponse to the command"
            # "command respond"
            n136 = Unbundle By Name(w396) -> ("Dependencies.RemoteControl"=w401:refnum<class "RemoteControl.lvclass">, "Self Reference"=w395:refnum<class "Instrument.lvclass">, "Message.Command"=w391:string, "Message.Data"=w398:variant, "Message.Message ID"=w399:i32)  [unwired: 1 out]
            "Remote Command" <- w391
            n137 = call-dynamic "Handle Command.vi"("error in (no error)"=w400, "Data"=w398, "Command"=w391, "Instrument in"=w395) -> ("error out"=w393:errorcluster, "Processed Data"=w397:variant, "Command"=w392:string)  [unwired: 4 in, 1 out]
            n138 = case shown="Default" w392 {
              selector: w392 -> [w405 _]
              tunnel: w401 -> [w410 _]
              tunnel: w393 -> [w411 w413]
              tunnel: w397 -> [w407 _]
              tunnel: w399 -> [w409 _]
              tunnel: [w406 w413] -> w394
              frame Default {
                n139 = Bundle By Name(cluster=T5 {"Message"={"Command"="", "Data"=variant(bool FALSE), "Message ID"=0}} ("SendMessgaeToProcess"), "Message.Command"=w405, "Message.Data"=w407, "Message.Message ID"=w409) -> (w408:T5)
                n140 = call "RemoteControl.SendMessageToProcess.vi"("error in (no error)"=w411, "SendMessageToProcess"=w408, "RemoteControl"=w410) -> ("error out"=w406:errorcluster)  [unwired: 7 in, 1 out]
              }
              frame "" {
              }
            }
            n141 = call <vilib>:"Add State(s) to Queue__jki_lib_state_machine.vi"("State(s) in (\"\")"=w404) -> ("States Out"=w403:string)  [unwired: 14 in]
          }
          frame "Instrument: Handle Local Command" {
            # "#todo\nput driver stuff inside this one"
            # "do stuff in reponse to the command"
            # "command respond"
            n142 = Unbundle By Name(w423) -> ("Self Reference"=w422:refnum<class "Instrument.lvclass">, "Message.Command"=w415:string, "Message.Data"=w424:variant, "Message.Message ID"=w414:i32)
            "Local Command" <- w415
            n143 = call-dynamic "Handle Command.vi"("error in (no error)"=w425, "Data"=w424, "Command"=w415, "Instrument in"=w422) -> ("error out"=w420:errorcluster, "Processed Data"=w417:variant, "Command"=w416:string, "Instrument out"=w418:refnum<class "Instrument.lvclass">)  [unwired: 4 in]
            n144 = case shown="Default" w416 {
              selector: w416 -> [_ w431]
              tunnel: [w429 w435] -> w421
              tunnel: w420 -> [w429 w434]
              tunnel: w418 -> [_ w433]
              tunnel: w417 -> [_ w432]
              tunnel: w414 -> [_ w430]
              frame "" {
              }
              frame Default {
                n145 = call "Instrument.MessageFromProcess.vi"("Message ID"=w430, "error in (no error)"=w434, "Message.Data"=w432, "Message.Command"=w431, "Instrument"=w433) -> ("error out"=w435:errorcluster)  [unwired: 5 in, 1 out]
              }
            }
            n146 = call <vilib>:"Add State(s) to Queue__jki_lib_state_machine.vi"("State(s) in Front (\"\")"="" ("State(s) in Front (\"\")"), "State(s) in (\"\")"=w428) -> ("States Out"=w427:string)  [unwired: 13 in]
          }
          frame "Instrument: getAll" {
            # "do this and can change dynamically\n(after running Inst Open for example)"
            # "get all parameters from the instrument"
            n147 = Unbundle By Name(w439) -> ("Self Reference"=w445:refnum<class "Instrument.lvclass">)
            n148 = call-dynamic "Handle Command.vi"("error in (no error)"=w446, "Command"="getAll", "Instrument in"=w445) -> ("error out"=w444:errorcluster, "Processed Data"=w437:variant, "Command"=w441:string, "Instrument out"=w440:refnum<class "Instrument.lvclass">)  [unwired: 5 in]
            n149 = case shown="Default" w441 {
              selector: w441 -> [w456 _]
              tunnel: w437 -> [w451 _]
              tunnel: w444 -> [w455 w459]
              tunnel: [w452 w459] -> w443
              tunnel: w440 -> [w457 _]
              tunnel: [w450 "" ("Paths")] -> w436
              frame Default {
                # "broadcast update to\nsubscribers (UI. Could be logger)"
                # "call data logger SMO"
                n150 = call "Instrument.MessageFromProcess.vi"("error in (no error)"=w455, "Message.Data"=w451, "Message.Command"=w456, "Instrument"=w457) -> ("error out"=w453:errorcluster, "Instrument out"=w454:refnum<class "Instrument.lvclass">)  [unwired: 6 in]
                n151 = call-dynamic "Get SMO PGSQL Log Paths.vi"("error in (no error)"=w453, "Instrument in"=w454) -> ("error out"=w452:errorcluster, "Paths"=w450:string)  [unwired: 7 in, 1 out]
              }
              frame "" {
                # "do nothing if command is empty"
              }
            }
            n152 = Bundle By Name(cluster=w439, "getAll"=w437, "Message.Data"=w437, "PGSQL.Address"=w436) -> (w438:T10)
            n153 = call <vilib>:"Add State(s) to Queue__jki_lib_state_machine.vi"("State(s) in (\"\")"=w449) -> ("States Out"=w448:string)  [unwired: 14 in]
          }
          frame "Instrument: Log to PGSQL" {
            # "send event to PGSQL process"
            n154 = Unbundle By Name(w462) -> ("Dependencies.Logger.PGSQL"=w465:refnum<class "Logger.PGSQL.lvclass">, "PGSQL.Address"=w461:string, "Message.Data"=w460:variant)
            n155 = call "Logger.PGSQL.WriteVariable.vi"("error in (no error)"=w464, "Data"=w460, "Address"=w461, "Logger"=w465) -> ("error out"=w463:errorcluster)  [unwired: 6 in, 1 out]
            n156 = call <vilib>:"Add State(s) to Queue__jki_lib_state_machine.vi"("State(s) in (\"\")"=w468) -> ("States Out"=w467:string)  [unwired: 14 in]
          }
          frame "Instrument: Open" {
            n157 = Unbundle By Name(w470) -> ("Self Reference"=w473:refnum<class "Instrument.lvclass">)
            n158 = call-dynamic "Open Instrument.vi"("error in (no error)"=w474, "Instrument in"=w473) -> ("error out"=w472:errorcluster, "Instrument out"=w471:refnum<class "Instrument.lvclass">)  [unwired: 8 in]
            n159 = Bundle By Name(cluster=w470, "Self Reference"=w471) -> (w469:T10)
            n160 = call <vilib>:"Add State(s) to Queue__jki_lib_state_machine.vi"("State(s) in (\"\")"=w477) -> ("States Out"=w476:string)  [unwired: 14 in]
          }
          frame "Instrument: Close" {
            n161 = Unbundle By Name(w479) -> ("Self Reference"=w482:refnum<class "Instrument.lvclass">)
            n162 = call-dynamic "Close Instrument.vi"("error in (no error)"=w483, "Instrument in"=w482) -> ("error out"=w481:errorcluster, "Instrument out"=w480:refnum<class "Instrument.lvclass">)  [unwired: 8 in]
            n163 = Bundle By Name(cluster=w479, "Self Reference"=w480) -> (w478:T10)
            n164 = call <vilib>:"Add State(s) to Queue__jki_lib_state_machine.vi"("State(s) in (\"\")"=w486) -> ("States Out"=w485:string)  [unwired: 14 in]
          }
        }
      }
    }
    frame Error {
    }
  }
  n165 = call-parent "Process.vi"("error in"=w7, "SMO"=w6) -> ("error out"=w4:errorcluster, "SMO out"=→"Instrument out":refnum<class "Instrument.lvclass">)  [unwired: 8 in]
  n166 = Merge Errors(w4, w3) -> (→"error out":errorcluster)
